vi "Find Item Type.vi"(0 "Directory Item in":string) -> (1 "Directory?":bool, 2 "Item Name":string, 3 "Item Size":u64)   [LabVIEW 2020, in "AoC 2022.lvlib"]
uses:
  AoC 2022.lvlib
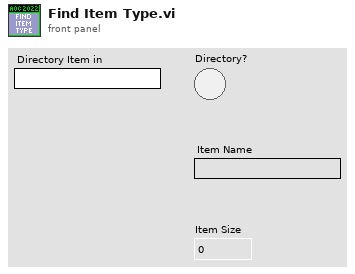
[diagram p1: front panel]
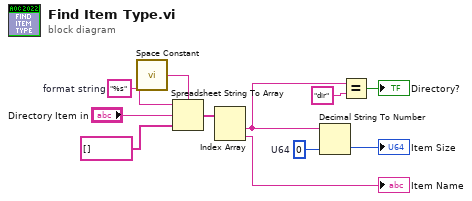
[diagram p0: block diagram]
diagram:
  w1 = u64 0  # U64
  w9 = "%s"  # format string
  n1 = call <vilib>:"Space Constant.vi"() -> ("String"=w11:string)
  n2 = Spreadsheet String To Array(delimiter (Tab)=w11, format string=w9, spreadsheet string="Directory Item in", array type (2D Dbl)=string[] []) -> (array=w7:string[])
  n3 = Index Array(array=w7) -> (element #1=w3:string, element #2=→"Item Name":string)  [unwired: 2 in]
  n4 = Decimal String To Number(string=w3, default (0L)=w1) -> (number=→"Item Size":u64)  [unwired: 1 in, 1 out]
  n5 = Equal?(x=w3, y="dir") -> (x = y?=→"Directory?":bool)
